vi "-8007 PCAN_ERROR_QXMTFULL Transmit queue is full--error.vi"(8 "error in":errorcluster, 11 "Channel":string) -> (0 "error out":errorcluster, 2 "Error Code":i32)   [LabVIEW 2018, in "PCANBasic.lvlib"]
uses:
  PCANBasic.lvlib
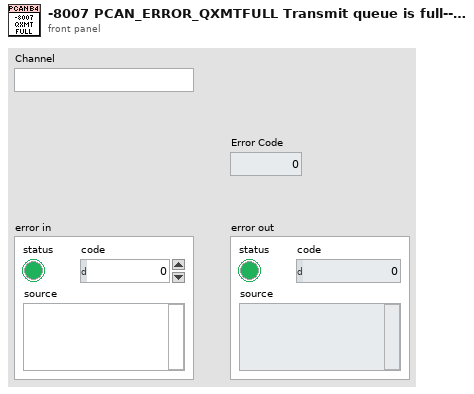
[diagram p1: front panel]
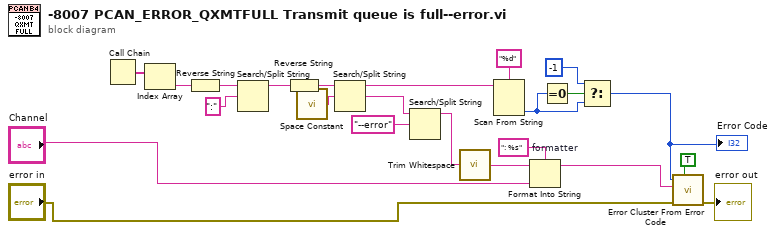
[diagram p0: block diagram]
diagram:
  w20 = ": %s"  # formatter
  n1 = Call Chain() -> (call chain=w15:string[])
  n2 = Index Array(array=w15) -> (element=w9:string)  [unwired: 1 in]
  n3 = Reverse String(1:w9) -> (0:w14:string)
  n4 = Search/Split String(string=w14, search string/char (-)=":") -> (substring before match=w13:string)  [unwired: 1 in, 2 out]
  n5 = Reverse String(1:w13) -> (0:w11:string)
  n6 = call <vilib>:"Space Constant.vi"() -> ("String"=w10:string)
  n7 = Search/Split String(string=w11, search string/char (-)=w10) -> (substring before match=w8:string, match + rest of string=w6:string)  [unwired: 1 in, 1 out]
  n8 = Search/Split String(string=w6, search string/char (-)="--error") -> (substring before match=w5:string)  [unwired: 1 in, 2 out]
  n9 = call <vilib>:"Trim Whitespace.vi"("string"=w5) -> ("trimmed string"=w4:string)  [unwired: 1 in]
  n10 = Scan From String(format string="%d", input string=w8) -> (output 1=w17:i32)  [unwired: 3 in, 3 out]
  n11 = Format Into String(format string=w20, initial string=w4, "Channel") -> (resulting string=w2:string)  [unwired: 1 in, 1 out]
  n12 = Equal To 0?(x=w17) -> (x = 0?=w18:bool)
  n13 = Select(t=-1, s=w18, f=w17) -> (s? t:f=w1:i32)
  "Error Code" <- w1
  n14 = call <vilib>:"Error Cluster From Error Code.vi"("show call chain? (False)"=TRUE, "error in (no error)"="error in", "error message (\"\")"=w2, "error code (0)"=w1) -> ("error out"=→"error out":errorcluster)  [unwired: 5 in]
